vi "Global_CMD_ACT_Data In.vi"() -> ()   [LabVIEW 2020, in "Shooter_ACT.lvlib"]
uses:
  roboRIO Code/Systems/Shooter/Shooter_ACT.lvlib
  Cluster_CMD_ACT_Data.ctl
  roboRIO Code/Systems/Shooter/ENUM_Shooter_Mode.ctl
panel:
  in  "CMD_ACT_Shooter_Data":T1
  # "The Names of the Data items in the Global Variable MUST describe who the Single Writer is\nFor Command Globals the Commander(CMD) represents Teleop or Autonomous or other command loop.\nThe naming convention for a Command Actuator Global is:   \n\nCMD_ACT_SubSystem_Data Name\n\nExample:\nCMD_ACT_Drive_Data\nCMD_ACT_Hopper_Eject Ball"
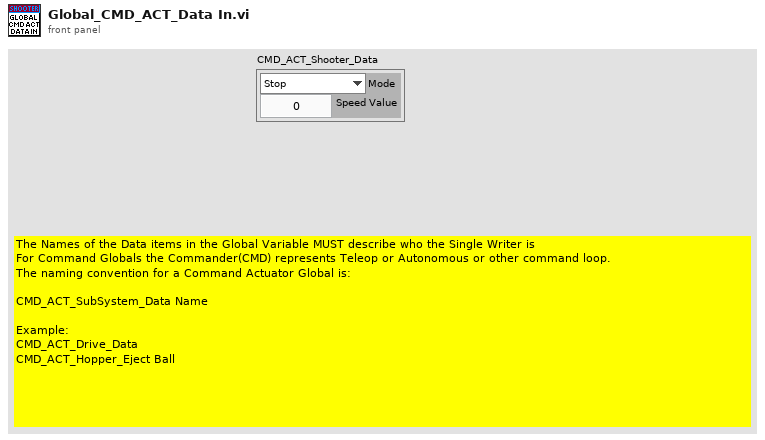
[diagram p1: front panel]
types:
  T1 = typedef "Shooter_ACT.lvlib/Cluster_CMD_ACT_Data.ctl" = cluster{"Mode":T2, "Speed Value":dbl}
  T2 = typedef "Shooter_ACT.lvlib/ENUM_Shooter_Mode.ctl" = enum16{"Stop", "Speed Percent", "Speed RPM"}
diagram:
